vi "Op-Trigger Output.vi"(8 "error in (no error)":errorcluster, 10 "trigger signal":i32(slide) scale=0.0..3.0, 11 "VISA session":refnum<visa-resource-name>) -> (0 "error out":errorcluster, 3 "VISA resource name out":refnum<visa-resource-name>)   [LabVIEW 2016, in "Agilent 415X Series.lvlib"]
doc: "This VI causes the instrument to send a trigger signal from its Ext. Trig. Out BNC connector. The selectable trigger signals are\n - Level High\n - Level Low\n - Positive Pulse\n - Negative Pulse"
uses:
  Agilent 415X Series.lvlib
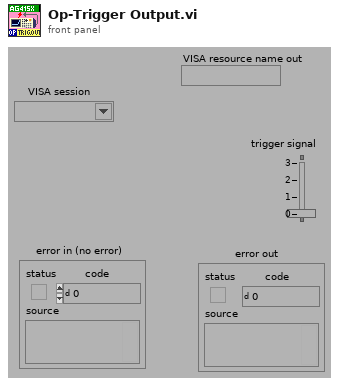
[diagram p1: front panel]
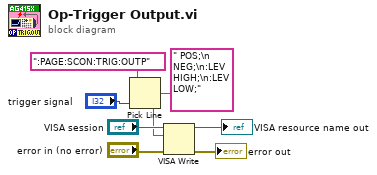
[diagram p0: block diagram]
diagram:
  n1 = Pick Line(string ("")=":PAGE:SCON:TRIG:OUTP", multi-line string=" POS;\n NEG;\n:LEV HIGH;\n:LEV LOW;", line index="trigger signal") -> (output string=w4:string)
  n2 = VISA Write(VISA resource name="VISA session", write buffer=w4, error in (no error)="error in (no error)") -> (VISA resource name out=→"VISA resource name out":refnum<visa-resource-name>, error out=→"error out":errorcluster)  [unwired: 1 out]
